vi "Insert Array Element.vi"(4 "Insert":string, 5 "Key name":string, 6 "Index":i32=4, 7 "Section name":string, 8 "error in (no error)":errorcluster, 9 "Use Key Regex? [F]":bool, 10 "Use Section Regex? [F]":bool, 11 "Carya Config in":refnum<class "Carya Config.lvclass">) -> (0 "error out":errorcluster, 3 "Carya Config out":refnum<class "Carya Config.lvclass">)   [LabVIEW 2013, in "Carya Config.lvclass"]
doc: "Copyright 2018, Carya Automatisering, Wiebe Walstra."
uses:
  Carya Config.lvclass
  CConfig Object/Search Replace Query/Search Replace Query.lvclass
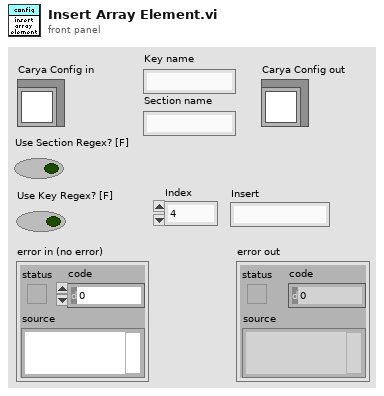
[diagram p1: front panel]
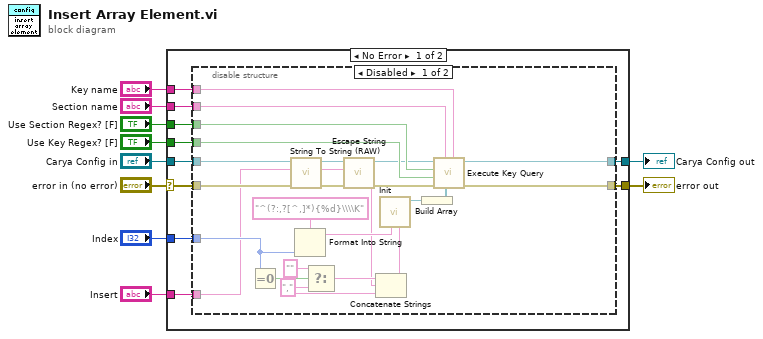
[diagram p0: block diagram]
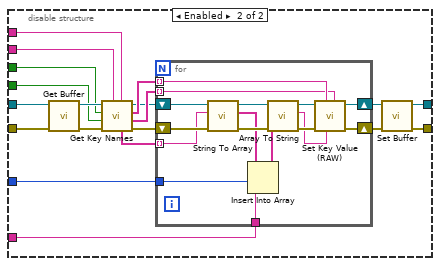
[diagram p2: hidden frame]
diagram:
  n1 = case shown="No Error" "error in (no error)" {
    selector: "error in (no error)" -> [w20 w82]
    tunnel: [w19 w82] -> w9
    tunnel: [w18 w81] -> w7
    tunnel: "Carya Config in" -> [w12 w81]
    tunnel: "Section name" -> [w15 _]
    tunnel: "Key name" -> [w14 _]
    tunnel: "Use Section Regex? [F]" -> [w17 _]
    tunnel: "Use Key Regex? [F]" -> [w16 _]
    tunnel: "Index" -> [w13 _]
    tunnel: "Insert" -> [w11 _]
    frame No Error {
      n2 = disable-structure shown="Disabled" {
        disable-tunnel: w20 -> [w45 w50]
        disable-tunnel: [w44 w48] -> w19
        disable-tunnel: [w43 w49] -> w18
        disable-tunnel: w17 -> [w42 w53]
        disable-tunnel: w16 -> [w41 w52]
        disable-tunnel: w15 -> [w40 w54]
        disable-tunnel: w14 -> [w39 w55]
        disable-tunnel: w13 -> [w33 w47]
        disable-tunnel: w12 -> [w26 w51]
        disable-tunnel: w11 -> [w23 w46]
        frame Disabled {
          w21 = "," ("f")
          n3 = Equal To 0?(x=w33) -> (x = 0?=w32:bool)
          n4 = call-dynamic "String To String (RAW).vi"("error in (no error)"=w45, "String"=w23, "Registry Object"=w26) -> ("error out"=w27:errorcluster, "String (RAW)"=w24:string, "Registry Object"=w25:refnum<class "Carya Config.lvclass">)  [unwired: 6 in]
          n5 = Format Into String(format string="^(?:,?[^,]*){%d}\\\\K" ("Regex"), w33) -> (resulting string=w35:string)  [unwired: 2 in, 1 out]
          n6 = Select(t="", s=w32, f=w21) -> (s? t:f=w30:string)
          n7 = call-dynamic "Escape String.vi"("error in (no error)"=w27, "String"=w24, "Registry Object"=w25) -> ("error out"=w29:errorcluster, "Escaped string"=w22:string, "Registry Object"=w28:refnum<class "Carya Config.lvclass">)  [unwired: 6 in]
          n8 = Concatenate Strings(w30, w22, w21) -> (w36:string)
          n9 = call "Init.vi"("Replace"=w36, "Search"=w35) -> ("Find First Query out"=w38:refnum<class "Search Replace Query.lvclass">)  [unwired: 8 in, 1 out]
          n10 = Build Array(w38) -> (w37:refnum<class "Search Replace Query.lvclass">[])
          n11 = call-dynamic "Execute Key Query.vi"("Key name"=w39, "Key queries"=w37, "Section name"=w40, "error in (no error)"=w29, "Use Key Regex? [F]"=w41, "Use Section Regex? [F]"=w42, "Carya Config in"=w28) -> ("error out"=w44:errorcluster, "Carya Config out"=w43:refnum<class "Carya Config.lvclass">)  [unwired: 2 in, 1 out]
        }
        frame Enabled {
          n12 = call-dynamic "Get Buffer.vi"("error in (no error)"=w50, "Carya Config in"=w51) -> ("error out"=w56:errorcluster, "Config"=w57:refnum<class "Carya Config.lvclass">)  [unwired: 8 in]
          n13 = call-dynamic "Get Key Names.vi"("Key name/Regex"=w55, "Section name/Regex"=w54, "error in (no error)"=w56, "Use Key Regex? [F]"=w52, "Use Section Regex? [F]"=w53, "Carya Config in"=w57) -> ("error out"=w61:errorcluster, "Key names"=w64:string[], "Section names"=w63:string[], "Carya Config out"=w59:refnum<class "Carya Config.lvclass">, "Context (concatenated)"=w62:string[])  [unwired: 1 in]
          n14 = for {
            shift-right: [w79] -> w60
            shift-left: w59 -> [w76]
            shift-right: [w80] -> w58
            shift-left: w61 -> [w78]
            tunnel: w62 -> [w75] mode=indexing
            tunnel: w63 -> [w69] mode=indexing
            tunnel: w64 -> [w68] mode=indexing
            tunnel: w47 -> [w67]
            tunnel: w46 -> [w65]
            n15 = call-dynamic "String To Array.vi"("error in (no error)"=w78, "resulting string"=w75, "Registry Object"=w76) -> ("error out"=w77:errorcluster, "Array"=w66:string[], "Registry Object"=w73:refnum<class "Carya Config.lvclass">)  [unwired: 6 in]
            n16 = Insert Into Array(array=w66, index=w67, new element=w65) -> (w71:string[])
            n17 = call-dynamic "Array To String.vi"("error in (no error)"=w77, "Array"=w71, "Registry Object"=w73) -> ("error out"=w74:errorcluster, "resulting string"=w70:string, "Registry Object"=w72:refnum<class "Carya Config.lvclass">)  [unwired: 6 in]
            n18 = call-dynamic "Set Key Value (RAW).vi"("Key name"=w68, "Key value"=w70, "Section name"=w69, "error in (no error)"=w74, "Carya Config in"=w72) -> ("error out"=w80:errorcluster, "Carya Config out"=w79:refnum<class "Carya Config.lvclass">)  [unwired: 2 in, 3 out]
          }
          n19 = call-dynamic "Set Buffer.vi"("error in (no error)"=w58, "Carya Config"=w60) -> ("error out"=w48:errorcluster, "Carya Config out"=w49:refnum<class "Carya Config.lvclass">)  [unwired: 8 in]
        }
      }
    }
    frame Error {
    }
  }
  "error out" <- w9
  "Carya Config out" <- w7
